vi "Decode Cordinate.vi"(10 "Encoded Cordinate":string) -> (2 "Decoded Cordinate":u32)   [LabVIEW 2022 SP3]
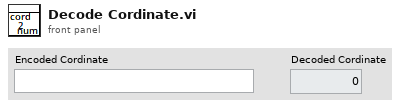
[diagram p1: front panel]
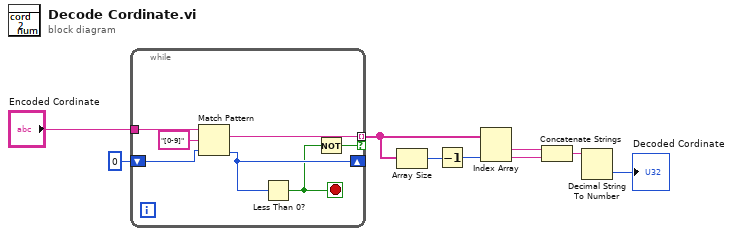
[diagram p0: block diagram]
diagram:
  n1 = while {
    tunnel: "Encoded Cordinate" -> [w16]
    tunnel: [w10] -> w7 mode=indexing if=w11
    shift-right: [w14] -> _
    shift-left: 0 ("offset past match") -> [w13]
    stop <- w12 stop-if-true
    n2 = Match Pattern(string=w16, regular expression="[0-9]", offset (0)=w13) -> (match substring=w10:string, offset past match=w14:i32)  [unwired: 2 out]
    n3 = Less Than 0?(x=w14) -> (x < 0?=w12:bool)
    n4 = Not(x=w12) -> (.not. x?=w11:bool)
  }
  n5 = Array Size(array=w7) -> (size(s)=w6:i32)
  n6 = Decrement(x=w6) -> (x-1=w5:i32)
  n7 = Index Array(array=w7, index #2=w5) -> (element #1=w4:string, element #2=w3:string)  [unwired: 1 in]
  n8 = Concatenate Strings(w4, w3) -> (w2:string)
  n9 = Decimal String To Number(string=w2) -> (number=→"Decoded Cordinate":i32)  [unwired: 2 in, 1 out]
